vi "initialise.vi"(8 "error in (no error)":errorcluster, 10 "writer buffer size":i32=100000 format="%.0e") -> (0 "error out":errorcluster, 2 "network streaming queues":T2, 3 "FPGA VI Reference Out":T1)   [LabVIEW 2010]
uses:
  network_streaming_queues_cluster.ctl
  type definitions/config_data_cluster.ctl
  type definitions/settings_cluster.ctl
  common_typedefs/channels_cluster.ctl
  type definitions/gate_cluster.ctl
  common_typedefs/gate_parameters_cluster.ctl
  FPGA_VI_reference.ctl
  <vilib>/userDefined/High Color/nirio_resource_hc.ctl
  type definitions/command_enum.ctl
  <vilib>/rvi/interface/nirviOpenFPGA/nirviOpenFPGA.xnode
  FPGA Bitfiles/PCIe-7842R_120MHz.lvbitx
  <vilib>/rvi/ClientSDK/nirviWhatTheDeviceIsDoing.ctl
  FPGA Bitfiles/PCIe-7842R_80MHz.lvbitx
  <vilib>/rvi/interface/nirviMethod/nirviMethod.xnode
  <vilib>/rvi/interface/nirviReadWriteControl/nirviReadWriteControl.xnode
  <vilib>/rvi/interface/common/niFpgaNodeNameForErrorReporting.ctl
  <vilib>/rvi/errors/niLvFpgaWhatHappensToTopLevelVI.ctl
  FPGA Bitfiles/PXI-7813R_80MHz.lvbitx
  FPGA Bitfiles/PXI-7813R_120MHz.lvbitx
  <vilib>/FPGAPlugInAG/PCIe-7842R/niLvFpga_Open_PCIe-7842R.vi
  <vilib>/rvi/interface/common/dynamic/niFpgaDynamicAddResources.vi
  <vilib>/FPGAPlugInAG/Dynamic/niLvFpga_Reset_Dynamic.vi
  <vilib>/Utility/error.llb/Error Cluster From Error Code.vi
  <vilib>/rvi/errors/niLvFpgaAdjustHostInterfaceError.vi
  <vilib>/FPGAPlugInAG/PXI-7813R/niLvFpga_Open_PXI-7813R.vi
  NiFpgaLv.dll
panel:
  out "FPGA VI Reference Out 3":T1
  in  "writer buffer size 3":i32=100000 format="%.0e"
  out "network streaming queues 3":T2
  out "error out 3":errorcluster
  in  "error in (no error) 3":errorcluster
  out "FPGA VI Reference Out 2":T1
  in  "writer buffer size 2":i32=100000 format="%.0e"
  out "network streaming queues 2":T2
  out "error out 2":errorcluster
  in  "error in (no error) 2":errorcluster
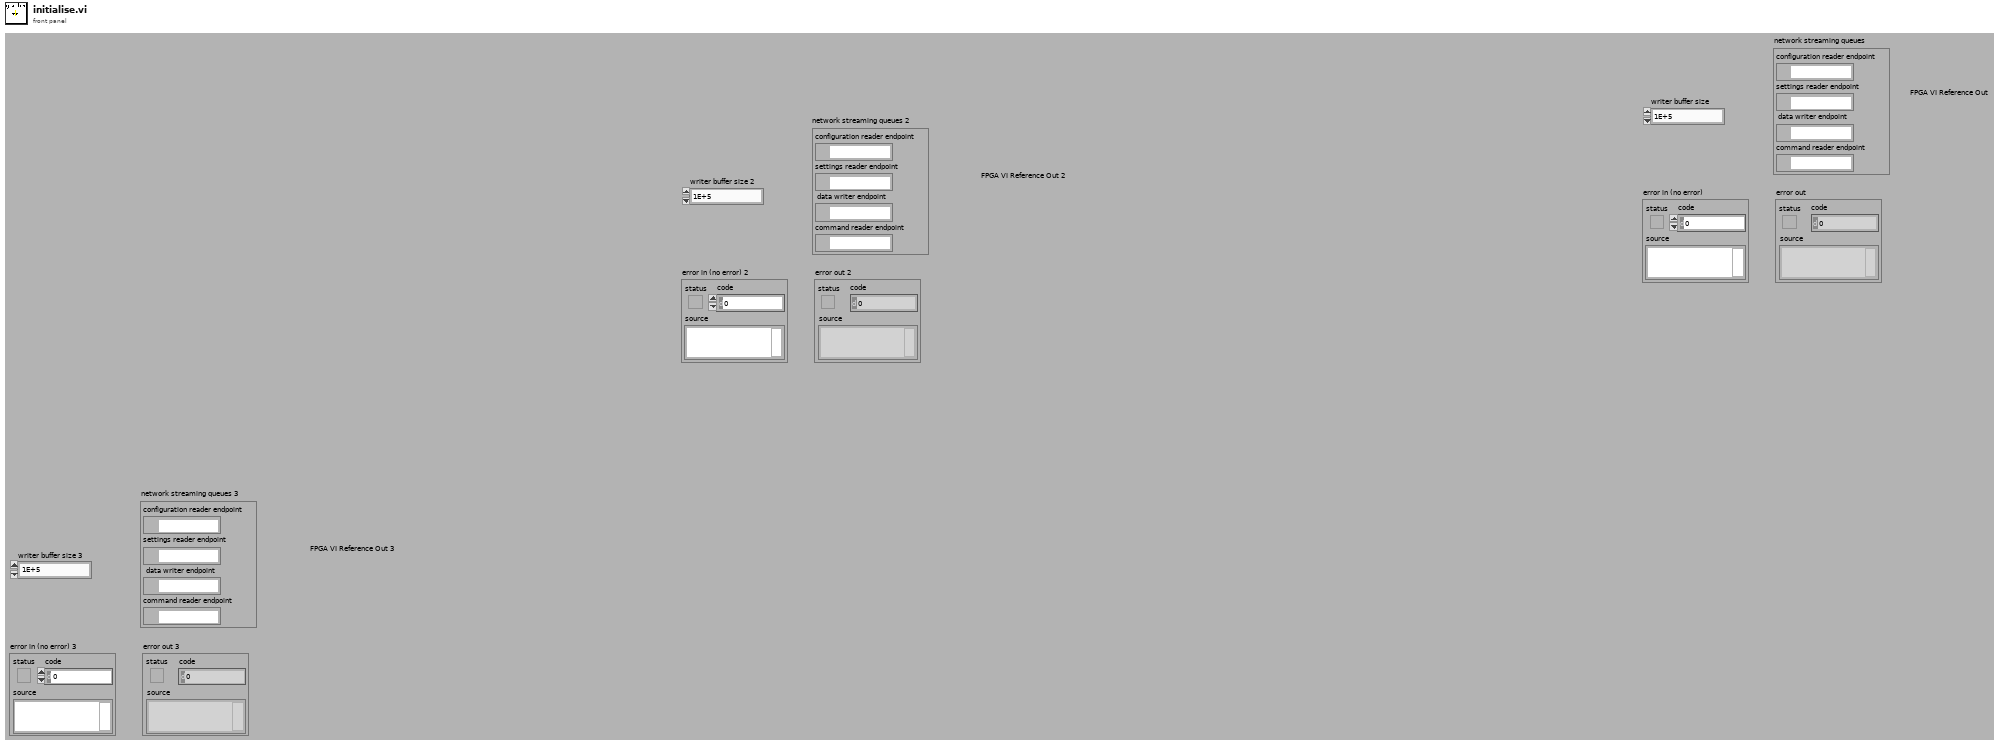
[diagram p1: front panel]
types:
  T1 = typedef "FPGA_VI_reference.ctl" = refnum<k20>
  T2 = typedef "network_streaming_queues_cluster.ctl" = cluster{"configuration reader endpoint":refnum<k21>, "settings reader endpoint":refnum<k21>, "data writer endpoint":refnum<k21>, "command reader endpoint":refnum<k21>}
  T3 = typedef "nirio_resource_hc.ctl" = tag
  T4 = enum32{"Invalid", "Standard", "Closed", "Hidden", "Minimized", "Maximized"}
  T5 = typedef "config_data_cluster.ctl" = cluster{"bit file":string, "hifo box version":i32, "ADC clock phase":i32}
  T6 = typedef "settings_cluster.ctl" = cluster{"number of pixels":i64, "pixel frequency (Hz)":dbl, "pixel values cluster":T7, "triggered?":bool, "triggered flag valid?":bool, "gates":T8[]}
  T7 = typedef "channels_cluster.ctl" = cluster{"channel 0":u32, "channel 1":u32, "channel 2":u32, "channel 3":u32}
  T8 = typedef "gate_cluster.ctl" = cluster{"index":i32, "parameters":T9}
  T9 = typedef "gate_parameters_cluster.ctl" = cluster{"offset":i64, "pulsing":i64, "not pulsing":i64, "cycles per pulse":i64, "repetitions":i64}
  T10 = typedef "command_enum.ctl" = enum16{"NULL", "update", "start", "stop", "reset", "shut-down"}
  T11 = typedef "nirviWhatTheDeviceIsDoing.ctl" = enum32{"nothing", "something other than LabVIEW FPGA", "FPGA interface", "interactive", "emulation"}
  T12 = typedef "niFpgaNodeNameForErrorReporting.ctl" = enum16{"Open FPGA VI Reference", "Read/Write Control", "Invoke Method: Abort", "Invoke Method: Acknowledge IRQ", "Invoke Method: Download", "Invoke Method: FIFO.Configure", "Invoke Method: FIFO.Read", "Invoke Method: FIFO.Start", "Invoke Method: FIFO.Stop", "Invoke Method: FIFO.Write", "Invoke Method: Reset", "Invoke Method: Run", "Invoke Method: Wait on IRQ", "Close FPGA VI Reference"}
  T13 = typedef "niLvFpgaWhatHappensToTopLevelVI.ctl" = enum16{"top level VI scripted behind XNode", "top level VI inlined behind XNode"}
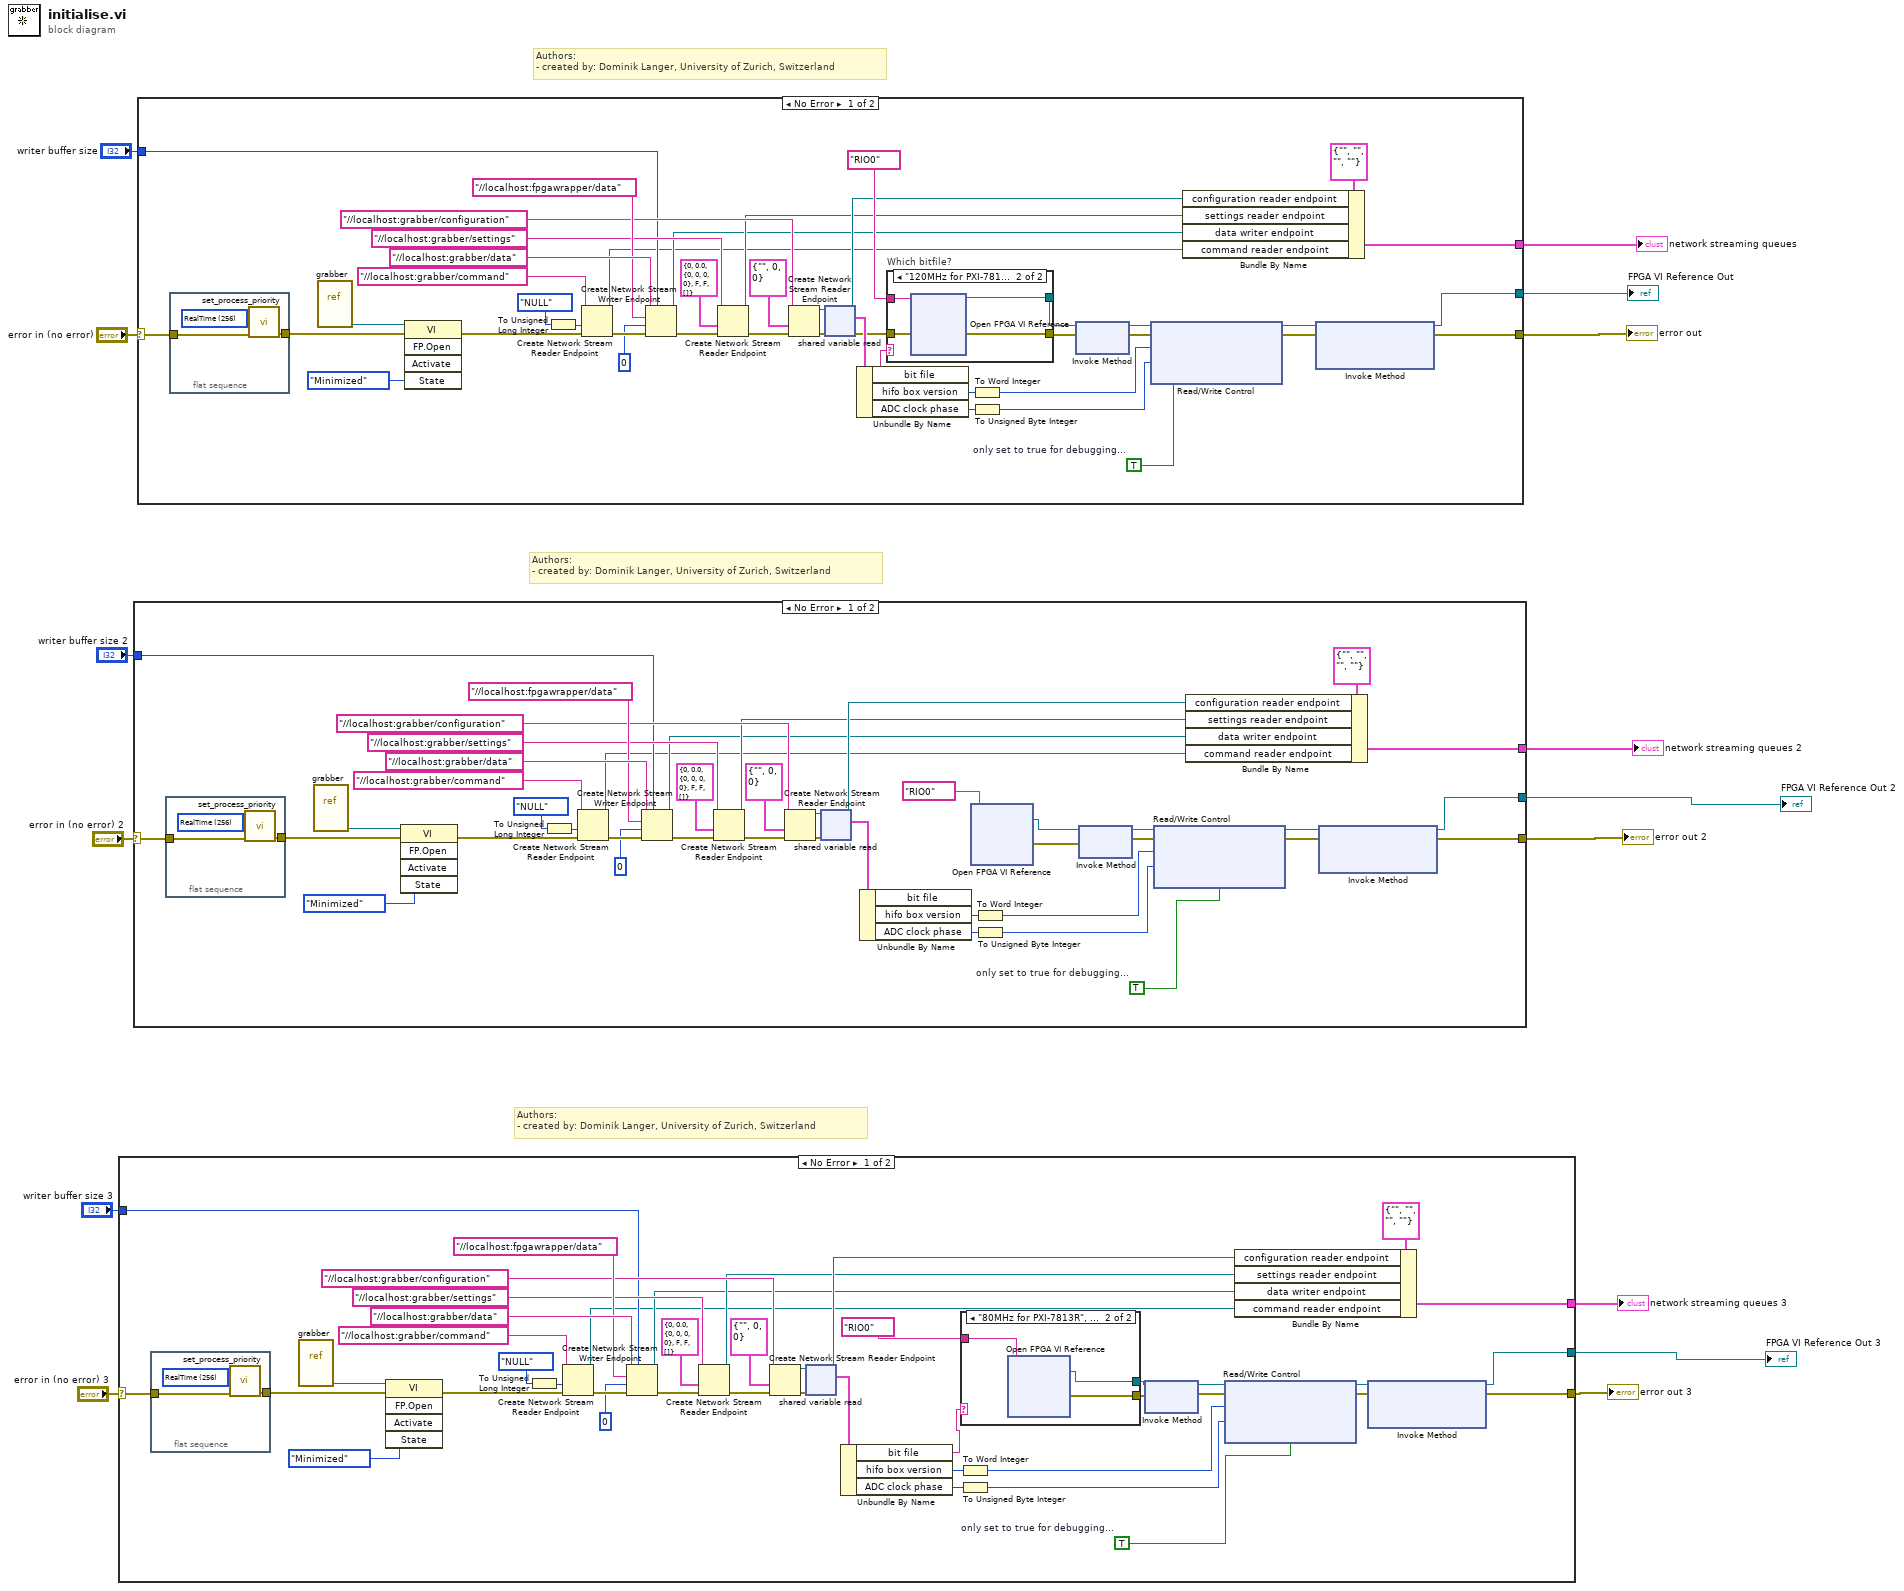
[diagram p0: block diagram]
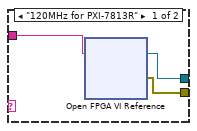
[diagram p2: hidden frame]
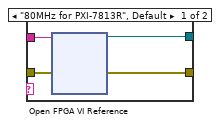
[diagram p5: hidden frame]
diagram:
  # "Authors: \n- created by: Dominik Langer, University of Zurich, Switzerland"
  # "Authors: \n- created by: Dominik Langer, University of Zurich, Switzerland"
  # "Authors: \n- created by: Dominik Langer, University of Zurich, Switzerland"
  n1 = case shown="No Error" "error in (no error) 3" {
    selector: "error in (no error) 3" -> [w33 w264]
    tunnel: [w32 w264] -> w4
    tunnel: "writer buffer size 3" -> [w31 _]
    tunnel: [w25 _] -> w2
    tunnel: [w24 _] -> w1
    frame No Error {
      w20 = TRUE  # only set to true for debugging...
      n2 = flat-sequence {
        tunnel: [w262] -> w22
        tunnel: w33 -> [w261]
        frame #0 {
          w263 = 256 items=["Normal"=32, "Idle"=64, "High"=128, "RealTime"=256, "BelowNormal"=16384, "AboveNormal"=32768] ("PriorityClass")
          n3 = call "set_process_priority.vi"("error in (no error)"=w261, "PriorityClass"=w263) -> ("error out"=w262:errorcluster)  [unwired: 9 in]
        }
      }
      n4 = vi-ref "grabber.vi"() -> (w23:refnum<vi>)
      n5 = invoke class="VI" method="FP.Open"(reference=w23, error in=w22, "State"=T4."Minimized") -> (error out=w21:errorcluster)  [unwired: 2 in, 4 out]
      n6 = To Unsigned Long Integer(number=command_enum."NULL" ("command")) -> (unsigned 32bit integer=w57:u32)
      n7 = Create Network Stream Reader Endpoint(8:w21, 9:w57, 11:"//localhost:grabber/command" ("writer name")) -> (0:w39:errorcluster, 3:w26:refnum<k21>)  [unwired: 3 in]
      n8 = Create Network Stream Writer Endpoint(7:w31, 8:w39, 9:u64 0, 10:"//localhost:fpgawrapper/data" ("reader url"), 11:"//localhost:grabber/data" ("writer name")) -> (0:w38:errorcluster, 3:w27:refnum<k21>)  [unwired: 1 in]
      n9 = Create Network Stream Reader Endpoint(8:w38, 9:T6 {"number of pixels"=0, "pixel frequency (Hz)"=0.0, "pixel values cluster"={"channel 0"=0, "channel 1"=0, "channel 2"=0, "channel 3"=0}, "triggered?"=FALSE, "triggered flag valid?"=FALSE, "gates"=[]} ("settings"), 11:"//localhost:grabber/settings" ("reader url")) -> (0:w41:errorcluster, 3:w28:refnum<k21>)  [unwired: 3 in]
      n10 = Create Network Stream Reader Endpoint(8:w41, 9:T5 {"bit file"="", "hifo box version"=0, "ADC clock phase"=0} ("config data"), 11:"//localhost:grabber/configuration" ("reader url")) -> (0:w53:errorcluster, 3:w52:refnum<k21>)  [unwired: 3 in]
      n11 = shared-variable-read(w52, w53) -> (w29:refnum<k21>, w45:T5)  [unwired: 1 in, 2 out]
      n12 = Unbundle By Name(w45) -> ("bit file"=w16:string, "hifo box version"=w44:i32, "ADC clock phase"=w43:i32)
      n13 = To Word Integer(number=w44) -> (16bit integer=w50:i16)
      n14 = To Unsigned Byte Integer(number=w43) -> (unsigned 8bit integer=w49:u8)
      n15 = case shown="\"80MHz for PXI-7813R\", Default" w16 {
        tunnel: [w60 w79] -> w19
        tunnel: [w59 w78] -> w18
        tunnel: T3 "RIO0" ("resource name") -> [w61 w77]
        frame "120MHz for PXI-7813R" {
          n16 = xnode "Open FPGA VI Reference"("resource name"=w61) -> ("FPGA VI Reference Out"=w60:refnum<k20>, "error out"=w59:errorcluster)  [unwired: 1 in]
        }
        frame "80MHz for PXI-7813R", Default {
          n17 = xnode "Open FPGA VI Reference"("resource name"=w77) -> ("FPGA VI Reference Out"=w79:refnum<k20>, "error out"=w78:errorcluster)  [unwired: 1 in]
        }
      }
      n18 = xnode "Invoke Method"("FPGA VI Reference In"=w19, "error in"=w18) -> ("FPGA VI Reference Out"=w51:refnum<k20>, "error out"=w48:errorcluster)
      n19 = xnode "Read/Write Control"("FPGA VI Reference In"=w51, "error in"=w48, "converter box version"=w50, "ADC clock phase"=w49, "clamp first pixel?"=w20) -> ("FPGA VI Reference Out"=w46:refnum<k20>, "error out"=w47:errorcluster)
      n20 = Bundle By Name(cluster=T2 {"configuration reader endpoint"="", "settings reader endpoint"="", "data writer endpoint"="", "command reader endpoint"=""} ("network streaming queues"), "configuration reader endpoint"=w29, "settings reader endpoint"=w28, "data writer endpoint"=w27, "command reader endpoint"=w26) -> (w25:T2)
      n21 = xnode "Invoke Method"("FPGA VI Reference In"=w46, "error in"=w47) -> ("FPGA VI Reference Out"=w24:refnum<k20>, "error out"=w32:errorcluster)  [unwired: 1 in]
    }
    frame Error {
    }
  }
  "error out 3" <- w4
  "network streaming queues 3" <- w2
  "FPGA VI Reference Out 3" <- w1
  n22 = case shown="No Error" "error in (no error) 2" {
    selector: "error in (no error) 2" -> [w281 w491]
    tunnel: [w280 w491] -> w9
    tunnel: "writer buffer size 2" -> [w279 _]
    tunnel: [w273 _] -> w7
    tunnel: [w272 _] -> w6
    frame No Error {
      w268 = TRUE  # only set to true for debugging...
      n23 = flat-sequence {
        tunnel: [w489] -> w270
        tunnel: w281 -> [w488]
        frame #0 {
          w490 = 256 items=["Normal"=32, "Idle"=64, "High"=128, "RealTime"=256, "BelowNormal"=16384, "AboveNormal"=32768] ("PriorityClass")
          n24 = call "set_process_priority.vi"("error in (no error)"=w488, "PriorityClass"=w490) -> ("error out"=w489:errorcluster)  [unwired: 9 in]
        }
      }
      n25 = vi-ref "grabber.vi"() -> (w271:refnum<vi>)
      n26 = invoke class="VI" method="FP.Open"(reference=w271, error in=w270, "State"=T4."Minimized") -> (error out=w269:errorcluster)  [unwired: 2 in, 4 out]
      n27 = To Unsigned Long Integer(number=command_enum."NULL" ("command")) -> (unsigned 32bit integer=w305:u32)
      n28 = Create Network Stream Reader Endpoint(8:w269, 9:w305, 11:"//localhost:grabber/command" ("writer name")) -> (0:w287:errorcluster, 3:w274:refnum<k21>)  [unwired: 3 in]
      n29 = Create Network Stream Writer Endpoint(7:w279, 8:w287, 9:u64 0, 10:"//localhost:fpgawrapper/data" ("reader url"), 11:"//localhost:grabber/data" ("writer name")) -> (0:w286:errorcluster, 3:w275:refnum<k21>)  [unwired: 1 in]
      n30 = Create Network Stream Reader Endpoint(8:w286, 9:T6 {"number of pixels"=0, "pixel frequency (Hz)"=0.0, "pixel values cluster"={"channel 0"=0, "channel 1"=0, "channel 2"=0, "channel 3"=0}, "triggered?"=FALSE, "triggered flag valid?"=FALSE, "gates"=[]} ("settings"), 11:"//localhost:grabber/settings" ("reader url")) -> (0:w289:errorcluster, 3:w276:refnum<k21>)  [unwired: 3 in]
      n31 = Create Network Stream Reader Endpoint(8:w289, 9:T5 {"bit file"="", "hifo box version"=0, "ADC clock phase"=0} ("config data"), 11:"//localhost:grabber/configuration" ("reader url")) -> (0:w301:errorcluster, 3:w300:refnum<k21>)  [unwired: 3 in]
      n32 = shared-variable-read(w300, w301) -> (w277:refnum<k21>, w293:T5)  [unwired: 1 in, 2 out]
      n33 = Unbundle By Name(w293) -> ("hifo box version"=w292:i32, "ADC clock phase"=w291:i32)  [unwired: 1 out]
      n34 = xnode "Open FPGA VI Reference"("resource name"=T3 "RIO0") -> ("FPGA VI Reference Out"=w266:refnum<k20>, "error out"=w265:errorcluster)  [unwired: 1 in]
      n35 = To Word Integer(number=w292) -> (16bit integer=w298:i16)
      n36 = To Unsigned Byte Integer(number=w291) -> (unsigned 8bit integer=w297:u8)
      n37 = xnode "Invoke Method"("FPGA VI Reference In"=w266, "error in"=w265) -> ("FPGA VI Reference Out"=w299:refnum<k20>, "error out"=w296:errorcluster)
      n38 = xnode "Read/Write Control"("FPGA VI Reference In"=w299, "error in"=w296, "converter box version"=w298, "ADC clock phase"=w297, "clamp first pixel?"=w268) -> ("FPGA VI Reference Out"=w294:refnum<k20>, "error out"=w295:errorcluster)
      n39 = Bundle By Name(cluster=T2 {"configuration reader endpoint"="", "settings reader endpoint"="", "data writer endpoint"="", "command reader endpoint"=""} ("network streaming queues"), "configuration reader endpoint"=w277, "settings reader endpoint"=w276, "data writer endpoint"=w275, "command reader endpoint"=w274) -> (w273:T2)
      n40 = xnode "Invoke Method"("FPGA VI Reference In"=w294, "error in"=w295) -> ("FPGA VI Reference Out"=w272:refnum<k20>, "error out"=w280:errorcluster)  [unwired: 1 in]
    }
    frame Error {
    }
  }
  "error out 2" <- w9
  "network streaming queues 2" <- w7
  "FPGA VI Reference Out 2" <- w6
  n41 = case shown="No Error" "error in (no error)" {
    selector: "error in (no error)" -> [w506 w743]
    tunnel: [w505 w743] -> w14
    tunnel: "writer buffer size" -> [w504 _]
    tunnel: [w498 _] -> w12
    tunnel: [w497 _] -> w11
    frame No Error {
      w493 = TRUE  # only set to true for debugging...
      n42 = flat-sequence {
        tunnel: [w741] -> w495
        tunnel: w506 -> [w740]
        frame #0 {
          w742 = 256 items=["Normal"=32, "Idle"=64, "High"=128, "RealTime"=256, "BelowNormal"=16384, "AboveNormal"=32768] ("PriorityClass")
          n43 = call "set_process_priority.vi"("error in (no error)"=w740, "PriorityClass"=w742) -> ("error out"=w741:errorcluster)  [unwired: 9 in]
        }
      }
      n44 = vi-ref "grabber.vi"() -> (w496:refnum<vi>)
      n45 = invoke class="VI" method="FP.Open"(reference=w496, error in=w495, "State"=T4."Minimized") -> (error out=w494:errorcluster)  [unwired: 2 in, 4 out]
      n46 = To Unsigned Long Integer(number=command_enum."NULL" ("command")) -> (unsigned 32bit integer=w534:u32)
      n47 = Create Network Stream Reader Endpoint(8:w494, 9:w534, 11:"//localhost:grabber/command" ("writer name")) -> (0:w512:errorcluster, 3:w499:refnum<k21>)  [unwired: 3 in]
      n48 = Create Network Stream Writer Endpoint(7:w504, 8:w512, 9:u64 0, 10:"//localhost:fpgawrapper/data" ("reader url"), 11:"//localhost:grabber/data" ("writer name")) -> (0:w511:errorcluster, 3:w500:refnum<k21>)  [unwired: 1 in]
      n49 = Create Network Stream Reader Endpoint(8:w511, 9:T6 {"number of pixels"=0, "pixel frequency (Hz)"=0.0, "pixel values cluster"={"channel 0"=0, "channel 1"=0, "channel 2"=0, "channel 3"=0}, "triggered?"=FALSE, "triggered flag valid?"=FALSE, "gates"=[]} ("settings"), 11:"//localhost:grabber/settings" ("reader url")) -> (0:w514:errorcluster, 3:w501:refnum<k21>)  [unwired: 3 in]
      n50 = Create Network Stream Reader Endpoint(8:w514, 9:T5 {"bit file"="", "hifo box version"=0, "ADC clock phase"=0} ("config data"), 11:"//localhost:grabber/configuration" ("reader url")) -> (0:w530:errorcluster, 3:w529:refnum<k21>)  [unwired: 3 in]
      n51 = shared-variable-read(w529, w530) -> (w502:refnum<k21>, w520:errorcluster, w522:T5)  [unwired: 1 in, 1 out]
      n52 = Unbundle By Name(w522) -> ("bit file"=w519:string, "hifo box version"=w517:i32, "ADC clock phase"=w516:i32)
      n53 = case "Which bitfile?" shown="\"120MHz for PXI-7813R\"" w519 {
        tunnel: w520 -> [w539 w558]
        tunnel: [w538 w556] -> w518
        tunnel: T3 "RIO0" ("resource name") -> [w537 w557]
        tunnel: [w536 w555] -> w492
        frame "80MHz for PXI-7813R", Default {
          n54 = xnode "Open FPGA VI Reference"("error in"=w539, "resource name"=w537) -> ("FPGA VI Reference Out"=w536:refnum<k20>, "error out"=w538:errorcluster)
        }
        frame "120MHz for PXI-7813R" {
          n55 = xnode "Open FPGA VI Reference"("error in"=w558, "resource name"=w557) -> ("FPGA VI Reference Out"=w555:refnum<k20>, "error out"=w556:errorcluster)
        }
      }
      n56 = To Word Integer(number=w517) -> (16bit integer=w527:i16)
      n57 = To Unsigned Byte Integer(number=w516) -> (unsigned 8bit integer=w526:u8)
      n58 = xnode "Invoke Method"("FPGA VI Reference In"=w492, "error in"=w518) -> ("FPGA VI Reference Out"=w528:refnum<k20>, "error out"=w525:errorcluster)
      n59 = xnode "Read/Write Control"("FPGA VI Reference In"=w528, "error in"=w525, "converter box version"=w527, "ADC clock phase"=w526, "clamp first pixel?"=w493) -> ("FPGA VI Reference Out"=w523:refnum<k20>, "error out"=w524:errorcluster)
      n60 = Bundle By Name(cluster=T2 {"configuration reader endpoint"="", "settings reader endpoint"="", "data writer endpoint"="", "command reader endpoint"=""} ("network streaming queues"), "configuration reader endpoint"=w502, "settings reader endpoint"=w501, "data writer endpoint"=w500, "command reader endpoint"=w499) -> (w498:T2)
      n61 = xnode "Invoke Method"("FPGA VI Reference In"=w523, "error in"=w524) -> ("FPGA VI Reference Out"=w497:refnum<k20>, "error out"=w505:errorcluster)  [unwired: 1 in]
    }
    frame Error {
    }
  }
  "error out" <- w14
  "network streaming queues" <- w12
  "FPGA VI Reference Out" <- w11
